vi "factorial.vi"() -> ()   [LabVIEW 2018]
panel:
  in  "Operand":dbl
  in  "Operator":string(combo)
  out "Result":dbl
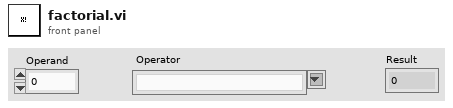
[diagram p1: front panel]
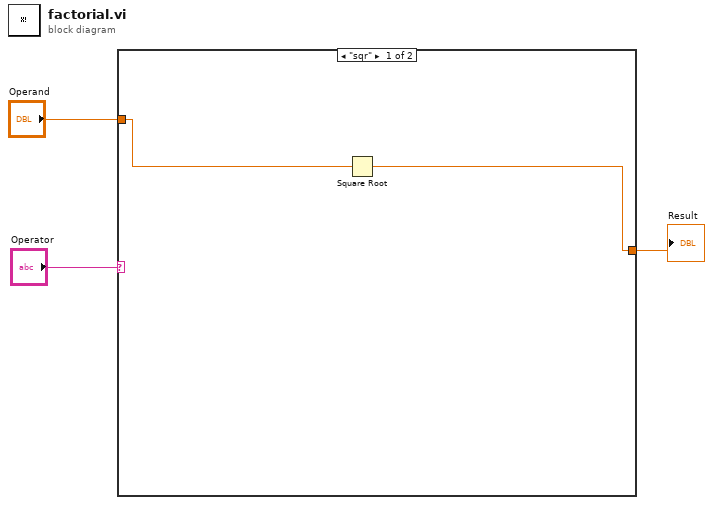
[diagram p0: block diagram]
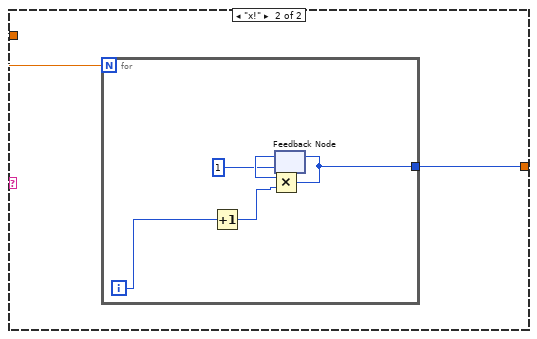
[diagram p2: hidden frame]
diagram:
  n1 = case shown="\"sqr\"" "Operator" {
    tunnel: "Operand" -> [w5 w7]
    tunnel: [w4 w6] -> w1
    frame "sqr" {
      n2 = Square Root(x=w5) -> (sqrt(x)=w4:dbl)
    }
    frame "x!" {
      n3 = for {
        N: w7 -> [_]
        tunnel: [w8] -> w6
        i -> [w9]
        n4 = Increment(x=w9) -> (x+1=w12:i32)
        n5 = feedback #1(1) -> (w11:i32)
        n6 = Multiply(x=w11, y=w12) -> (x*y=w8:i32)
        n7 = feedback-in #1(w8) -> ()
      }
    }
  }
  "Result" <- w1
